vi "Untitled 2.vi"() -> ()   [LabVIEW 2019]
uses:
  UI Actor.lvclass
  C:/Program Files/National Instruments/LabVIEW 2019/vi.lib/ActorFramework/Actor/Actor.lvclass
  UI Actor.lvclass/UI Actor.ctl
  Write Monedas.vi
  Write Productos.vi
  <vilib>/ActorFramework/Actor/Actor.lvclass
panel:
  in  "Productos":enum16{"Coca", "Nestle"}(ring)
  in  "Monedas":u16
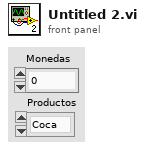
[diagram p1: front panel]
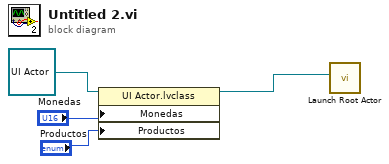
[diagram p0: block diagram]
diagram:
  n1 = property class="UI Actor.lvclass"(reference=refnum<class "UI Actor.lvclass"> refnum ("UI Actor.lvlib:UI Actor.lvclass"), "Monedas"="Monedas", "Productos"="Productos") -> (reference out=w3:refnum<class "UI Actor.lvclass">)  [unwired: 1 in, 1 out]
  n2 = call <vilib>:"Launch Root Actor.vi"("Actor"=w3) -> ()  [unwired: 9 in, 2 out]
